vi "Test Comm.vi"() -> ()   [LabVIEW 2021]
uses:
  CIFChannels/Typedef/Direction.ctl
  CIF_NIChn_Fifo_DAQ.lvclass
  D:/dev/CIF-LVCore/src/Channels/CIFChannels/CIFChannels.lvclass
  D:/dev/CIF-LVCore/src/Channels/CIF_NIChn/NIChn/CIF_NIChn.lvclass
  ChannelCommon/typedef/FIFO Config.ctl
  ChannelCommon/typedef/TimeStamps.ctl
  ChannelCommon/typedef/Datatype Waveform.ctl
  CIF_NIChn_Fifo_DAQ.lvclass/CIF_NIChn_Fifo_DAQ.ctl
  ChannelCommon/CIFFIFO/CIFfifo.lvclass/CIFfifo.ctl
  NIChn/CIF_NIChn.lvclass/CIF_NIChn.ctl
  CIFChannels/CIFChannels.lvclass/CIFChannels.ctl
  CIFCore/Common/Utilities/Add Error.vi
  SubVIs/Core Write DAQ FIFO.vi
  SubVIs/Core Read DAQ FIFO.vi
  CIFCore/Common/Utilities/Append Error Location.vi
  ChannelCommon/Utilities/Reset Waveform DVRs.vi
  SubVIs/Core Write DAQ DVR FIFO.vi
  ChannelCommon/Utilities/Get Waveform DVRs.vi
  SubVIs/Core Read DAQ DVR FIFO.vi
  <vilib>/CIFChannels/Top Level/Write Variable Length U8 Array.vi
  NIChn/Accessors/Read CIF Channel.vi
  NIChn/Accessors/Write CIF Channel.vi
  SubVIs/Flatten.vi
  ChannelCommon/CIFFIFO/Accessors/Read Length.vi
  NIChn/SubVIs/Check Disconnect.vi
  <vilib>/CIFChannels/Top Level/Read Variable Length U8 Array.vi
  SubVIs/Unflatten.vi
  CIFChannels/Accessors/Read Channel State.vi
  CIFChannels/Accessors/Read Direction.vi
  <vilib>/CIFChannels/SubVIs/Get dll Path.vi
  ChannelCommon/CIFFIFO/Utilities/Update Header.vi
  ChannelCommon/CIFFIFO/Flatten/DVR Flatten.vi
  ChannelCommon/CIFFIFO/Accessors/Write T0.vi
  ChannelCommon/CIFFIFO/Accessors/Write T_Out.vi
  ChannelCommon/CIFFIFO/Accessors/Write ClockID.vi
  CIFChannels/Accessors/Write Channel State.vi
  CIFChannels/Accessors/Read Disconnect Behavior.vi
  <vilib>/CIFChannels/Top Level/Read Variable Length U8 Array.vi/81056090-23cf-424a-a716-29db01c8ef1b.vi
  <vilib>/CIFChannels/Top Level/Read Variable Length U8 Array.vi/6610cd62-0a6d-4591-8fd4-6453482a4bc1.vi
  <vilib>/CIFChannels/Top Level/Read Variable Length U8 Array.vi/93d598b0-524b-4f76-9570-a74a86ef2c6f.vi
  ChannelCommon/CIFFIFO/Accessors/Write Timeout.vi
  ChannelCommon/CIFFIFO/Flatten/DVR Unflatten.vi
  ChannelCommon/CIFFIFO/Accessors/Read Header.vi
  ChannelCommon/CIFFIFO/Accessors/Write Header.vi
  ChannelCommon/Utilities/Flatten Header.vi
  ChannelCommon/CIFFIFO/Flatten/DVR Flatten.vi/6fdbece9-bad6-4a8e-9bf7-fe1528478dd6.vi
  ChannelCommon/CIFFIFO/Accessors/Write Payload Length.vi
  <vilib>/CIFChannels/Top Level/Read Variable Length U8 Array.vi/81056090-23cf-424a-a716-29db01c8ef1b.vi/4bc1c15b-36ab-481f-b8dd-c64075ce723a.vi
  <vilib>/CIFChannels/Top Level/Read Variable Length U8 Array.vi/81056090-23cf-424a-a716-29db01c8ef1b.vi/d83cb72b-7713-41fc-a3d1-682de79cf574.vi
  <vilib>/CIFChannels/Top Level/Read Variable Length U8 Array.vi/6610cd62-0a6d-4591-8fd4-6453482a4bc1.vi/c28b0ead-42ad-4072-80a2-aca7f2bd7ce3.vi
  <vilib>/CIFChannels/Top Level/Read Variable Length U8 Array.vi/93d598b0-524b-4f76-9570-a74a86ef2c6f.vi/4bc1c15b-36ab-481f-b8dd-c64075ce723a.vi
  <vilib>/CIFChannels/Top Level/Read Variable Length U8 Array.vi/93d598b0-524b-4f76-9570-a74a86ef2c6f.vi/d83cb72b-7713-41fc-a3d1-682de79cf574.vi
  ChannelCommon/Utilities/Unflatten Header.vi
  ChannelCommon/CIFFIFO/Flatten/DVR Flatten.vi/6fdbece9-bad6-4a8e-9bf7-fe1528478dd6.vi/c28b0ead-42ad-4072-80a2-aca7f2bd7ce3.vi
  NIChn/CIF_NIChn.lvclass
  ChannelCommon/Utilities/Update Time.vi
  ChannelCommon/ChannelCommon.lvlib
  CIFChannels/CIFChannels.lvclass
panel:
  out "status":string
  out "pass":bool
  out "error out":errorcluster
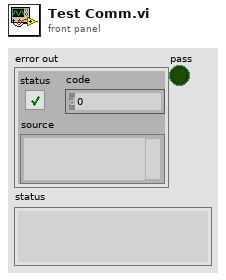
[diagram p1: front panel]
types:
  T1 = typedef "CIFChannels.lvclass/Direction.ctl" = enum16{"Publisher", "Subscriber"}
  T2 = typedef "ChannelCommon.lvlib/TimeStamps.ctl" = cluster{"ClockID":u8, "T0":u64, "T_Out":u64}
  T3 = typedef "ChannelCommon.lvlib/FIFO Config.ctl" = cluster{"Depth":u64, "Flags":u64, "ClockID":u8}
  T4 = typedef "ChannelCommon.lvlib/Datatype Waveform.ctl" = cluster{"measurement":dbl[], "dT":dbl, "Timestamp":u64, "Read Lock":bool}
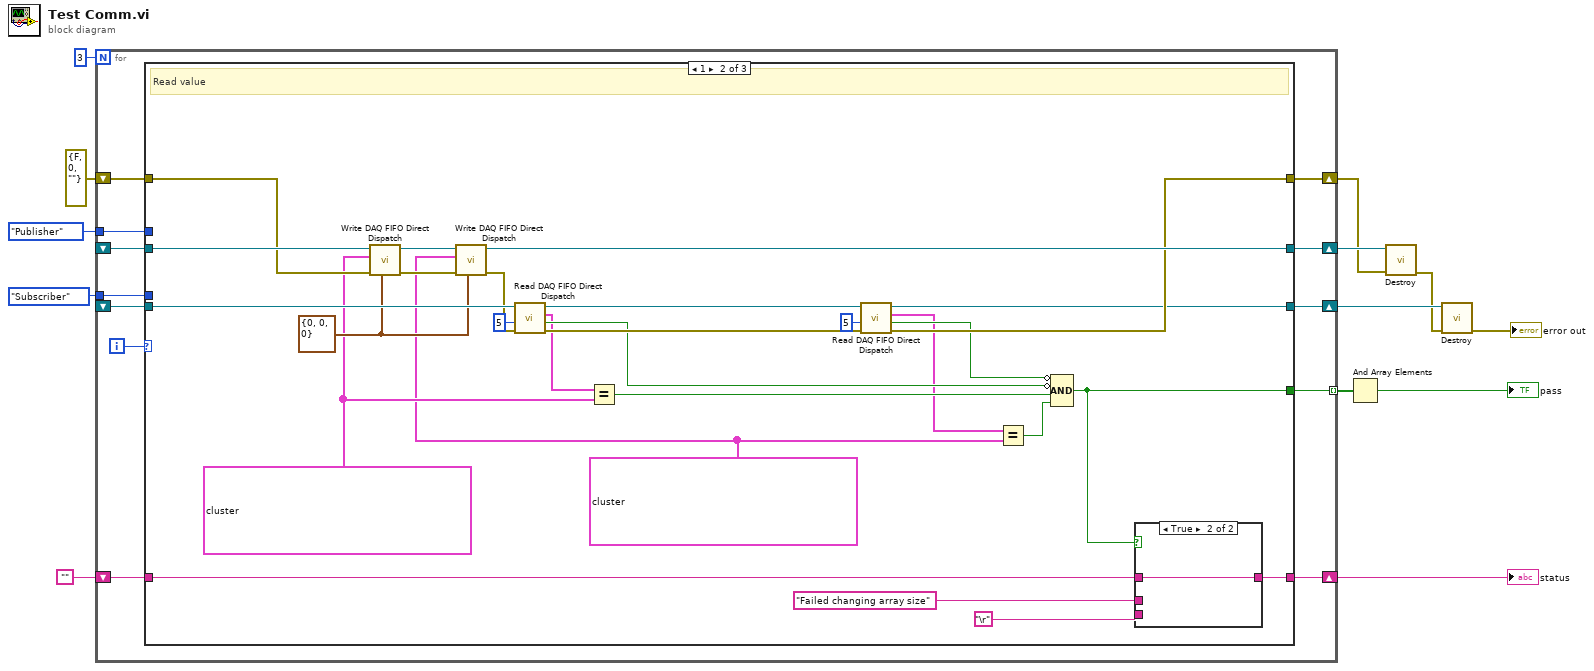
[diagram p0: block diagram]
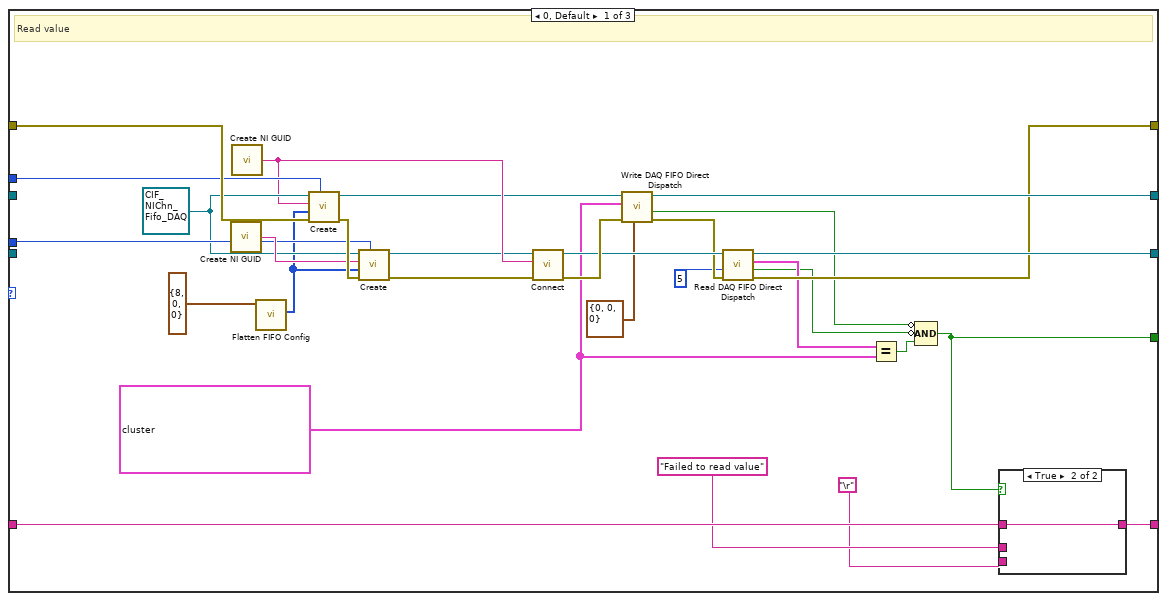
[diagram p2: hidden frame]
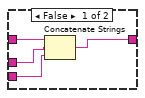
[diagram p3: hidden frame]
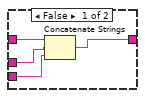
[diagram p4: hidden frame]
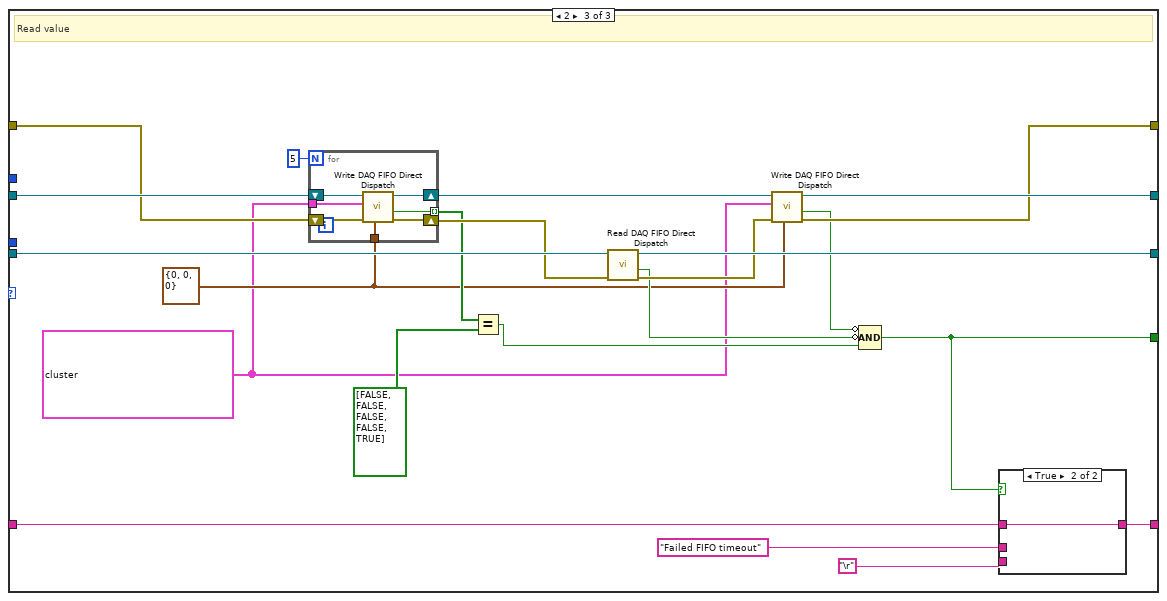
[diagram p5: hidden frame]
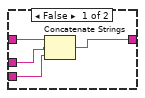
[diagram p6: hidden frame]
diagram:
  n1 = for {
    N: 3 -> [_]
    tunnel: [w25] -> w13 mode=indexing
    shift-right: [w23] -> w3
    shift-left: errorcluster {"status"=FALSE, "code"=0, "source"=""} ("error out") -> [w24]
    shift-right: [w20] -> w9
    shift-left: "" -> [w21]
    tunnel: Direction."Subscriber" ("Direction") -> [w19]
    tunnel: Direction."Publisher" ("Direction") -> [w18]
    shift-right: [w17] -> w5
    shift-left: _ -> [w15]
    shift-right: [w16] -> w4
    shift-left: _ -> [w14]
    i -> [w22]
    n2 = case shown="1" w22 {
      tunnel: [w50 w83 w95] -> w25
      tunnel: w24 -> [w48 w79 w109]
      tunnel: [w33 w72 w101] -> w23
      tunnel: w21 -> [w55 w87 w114]
      tunnel: [w54 w86 w113] -> w20
      tunnel: w19 -> [w46 _ _]
      tunnel: w18 -> [w45 _ _]
      tunnel: [w34 w69 w106] -> w17
      tunnel: [w36 w76 w104] -> w16
      tunnel: w14 -> [_ w80 w110]
      tunnel: w15 -> [_ w75 w107]
      frame 0, Default {
        w26 = T4[] [{"measurement"=array[986 elements], "dT"=43.0, "Timestamp"=2, "Read Lock"=FALSE}, {"measurement"=array[1001 elements], "dT"=34.0, "Timestamp"=1, "Read Lock"=FALSE}] ("DAQ In")
        w44 = refnum<class "CIF_NIChn_Fifo_DAQ.lvclass"> refnum ("CIF_NIChn_Fifo_Power.lvclass")
        # "Read value"
        n3 = call <vilib>:"Create NI GUID.vi"() -> ("NI GUID"=w47:string)
        n4 = call <vilib>:"Create NI GUID.vi"() -> ("NI GUID"=w41:string)
        n5 = call "Flatten FIFO Config.vi"("FIFO Config in"=T3 {"Depth"=8, "Flags"=0, "ClockID"=0}) -> ("Flattened Data out"=w42:u8[])  [unwired: 8 in, 2 out]
        n6 = call-dynamic "Create.vi"("Direction"=w45, "error in (no error)"=w48, "Custom Config Data"=w42, "Name"=w41, "CIFTag in"=w44) -> ("error out"=w49:errorcluster, "CIFTag out"=w38:refnum<class "CIF_NIChn_Fifo_DAQ.lvclass">)  [unwired: 5 in]
        n7 = call-dynamic "Create.vi"("Direction"=w46, "error in (no error)"=w49, "Custom Config Data"=w42, "Name"=w47, "CIFTag in"=w44) -> ("error out"=w40:errorcluster, "CIFTag out"=w39:refnum<class "CIF_NIChn_Fifo_DAQ.lvclass">)  [unwired: 5 in]
        n8 = call-dynamic "Connect.vi"("error in (no error)"=w40, "Connection Name"=w41, "CIFTag in"=w39) -> ("error out"=w37:errorcluster, "CIFTag out"=w35:refnum<class "CIF_NIChn_Fifo_DAQ.lvclass">)  [unwired: 7 in]
        n9 = call "Write DAQ FIFO Direct Dispatch.vi"("FIFO Timestamps"=T2 {"ClockID"=0, "T0"=0, "T_Out"=0}, "error in (no error)"=w37, "DAQ In"=w26, "CIFTag in"=w38) -> ("error out"=w32:errorcluster, "timed out?"=w31:bool, "CIFTag out"=w36:refnum<class "CIF_NIChn_Fifo_DAQ.lvclass">)  [unwired: 4 in, 1 out]
        n10 = call "Read DAQ FIFO Direct Dispatch.vi"("error in (no error)"=w32, "Timeout (ms)"=5, "CIFTag in"=w35) -> ("error out"=w33:errorcluster, "timed out?"=w29:bool, "DAQ Out"=w30:T4[], "CIFTag out"=w34:refnum<class "CIF_NIChn_Fifo_DAQ.lvclass">)  [unwired: 4 in, 1 out]
        n11 = Equal?(x=w30, y=w26) -> (x = y?=w51:bool)
        n12 = Compound Arithmetic op=AND(invert w31, invert w29, w51) -> (w50:bool)
        n13 = case shown="True" w50 {
          tunnel: w55 -> [w59 w60]
          tunnel: [w56 w60] -> w54
          tunnel: "Failed to read value" -> [w58 _]
          tunnel: "\r" -> [w57 _]
          frame False {
            n14 = Concatenate Strings(w59, w58, w57) -> (w56:string)
          }
          frame True {
          }
        }
      }
      frame 1 {
        w61 = T4[] [{"measurement"=array[986 elements], "dT"=213.0, "Timestamp"=2, "Read Lock"=FALSE}, {"measurement"=array[1001 elements], "dT"=32.0, "Timestamp"=1, "Read Lock"=FALSE}, {"measurement"=array[988 elements], "dT"=123.0, "Timestamp"=4, "Read Lock"=FALSE}] ("DAQ In")
        w62 = T4[] [{"measurement"=array[986 elements], "dT"=1.0, "Timestamp"=2, "Read Lock"=FALSE}, {"measurement"=array[1001 elements], "dT"=83.0, "Timestamp"=1, "Read Lock"=FALSE}, {"measurement"=array[988 elements], "dT"=78.0, "Timestamp"=4, "Read Lock"=FALSE}] ("DAQ In")
        w63 = T2 {"ClockID"=0, "T0"=0, "T_Out"=0} ("FIFO Timestamps")
        # "Read value"
        n15 = call "Write DAQ FIFO Direct Dispatch.vi"("FIFO Timestamps"=w63, "error in (no error)"=w79, "DAQ In"=w62, "CIFTag in"=w80) -> ("error out"=w77:errorcluster, "CIFTag out"=w78:refnum<class "CIF_NIChn_Fifo_DAQ.lvclass">)  [unwired: 4 in, 2 out]
        n16 = call "Write DAQ FIFO Direct Dispatch.vi"("FIFO Timestamps"=w63, "error in (no error)"=w77, "DAQ In"=w61, "CIFTag in"=w78) -> ("error out"=w73:errorcluster, "CIFTag out"=w76:refnum<class "CIF_NIChn_Fifo_DAQ.lvclass">)  [unwired: 4 in, 2 out]
        n17 = call "Read DAQ FIFO Direct Dispatch.vi"("error in (no error)"=w73, "Timeout (ms)"=5, "CIFTag in"=w75) -> ("error out"=w71:errorcluster, "timed out?"=w67:bool, "DAQ Out"=w64:T4[], "CIFTag out"=w68:refnum<class "CIF_NIChn_Fifo_DAQ.lvclass">)  [unwired: 4 in, 1 out]
        n18 = Equal?(x=w64, y=w62) -> (x = y?=w81:bool)
        n19 = call "Read DAQ FIFO Direct Dispatch.vi"("error in (no error)"=w71, "Timeout (ms)"=5, "CIFTag in"=w68) -> ("error out"=w72:errorcluster, "timed out?"=w66:bool, "DAQ Out"=w65:T4[], "CIFTag out"=w69:refnum<class "CIF_NIChn_Fifo_DAQ.lvclass">)  [unwired: 4 in, 1 out]
        n20 = Equal?(x=w65, y=w61) -> (x = y?=w82:bool)
        n21 = Compound Arithmetic op=AND(invert w66, invert w67, w81, w82) -> (w83:bool)
        n22 = case shown="True" w83 {
          tunnel: w87 -> [w91 w92]
          tunnel: [w88 w92] -> w86
          tunnel: "Failed changing array size" -> [w90 _]
          tunnel: "\r" -> [w89 _]
          frame False {
            n23 = Concatenate Strings(w91, w90, w89) -> (w88:string)
          }
          frame True {
          }
        }
      }
      frame 2 {
        w93 = T4[] [{"measurement"=array[986 elements], "dT"=43.0, "Timestamp"=2, "Read Lock"=FALSE}, {"measurement"=array[1001 elements], "dT"=34.0, "Timestamp"=1, "Read Lock"=FALSE}] ("DAQ In")
        w94 = T2 {"ClockID"=0, "T0"=0, "T_Out"=0} ("FIFO Timestamps")
        # "Read value"
        n24 = for {
          N: 5 -> [_]
          tunnel: w93 -> [w119]
          tunnel: w94 -> [w118]
          shift-right: [w117] -> w105
          shift-left: w110 -> [w121]
          tunnel: [w116] -> w100 mode=indexing
          shift-right: [w115] -> w103
          shift-left: w109 -> [w120]
          n25 = call "Write DAQ FIFO Direct Dispatch.vi"("FIFO Timestamps"=w118, "error in (no error)"=w120, "DAQ In"=w119, "CIFTag in"=w121) -> ("error out"=w115:errorcluster, "timed out?"=w116:bool, "CIFTag out"=w117:refnum<class "CIF_NIChn_Fifo_DAQ.lvclass">)  [unwired: 4 in, 1 out]
        }
        n26 = Equal?(x=w100, y=bool[] [FALSE, FALSE, FALSE, FALSE, TRUE]) -> (x = y?=w96:bool)
        n27 = call "Read DAQ FIFO Direct Dispatch.vi"("error in (no error)"=w103, "CIFTag in"=w107) -> ("error out"=w102:errorcluster, "timed out?"=w98:bool, "CIFTag out"=w106:refnum<class "CIF_NIChn_Fifo_DAQ.lvclass">)  [unwired: 5 in, 2 out]
        n28 = call "Write DAQ FIFO Direct Dispatch.vi"("FIFO Timestamps"=w94, "error in (no error)"=w102, "DAQ In"=w93, "CIFTag in"=w105) -> ("error out"=w101:errorcluster, "timed out?"=w97:bool, "CIFTag out"=w104:refnum<class "CIF_NIChn_Fifo_DAQ.lvclass">)  [unwired: 4 in, 1 out]
        n29 = Compound Arithmetic op=AND(invert w97, invert w98, w96) -> (w95:bool)
        n30 = case shown="True" w95 {
          tunnel: w114 -> [w125 w126]
          tunnel: [w122 w126] -> w113
          tunnel: "Failed FIFO timeout" -> [w124 _]
          tunnel: "\r" -> [w123 _]
          frame False {
            n31 = Concatenate Strings(w125, w124, w123) -> (w122:string)
          }
          frame True {
          }
        }
      }
    }
  }
  "status" <- w9
  n32 = And Array Elements(Boolean array=w13) -> (logical AND=→"pass":bool)
  n33 = call-dynamic "Destroy.vi"("error in (no error)"=w3, "CIF_NIChn_Fifo_Power_DVR in"=w4) -> ("error out"=w2:errorcluster)  [unwired: 8 in, 1 out]
  n34 = call-dynamic "Destroy.vi"("error in (no error)"=w2, "CIF_NIChn_Fifo_Power_DVR in"=w5) -> ("error out"=→"error out":errorcluster)  [unwired: 8 in, 1 out]
